vi "Acquire_Topology_Matrix.vi"(9 "All Path Array":string[](array[string]), 11 "Cluster of 7 Type Data":T2(array[cluster])) -> (2 "Topology Matrix":dbl[][](array[numeric]))   [LabVIEW 2014]
doc: "生成节点的拓扑矩阵"
uses:
  <vilib>/Analysis/Matrix/Datatypes/RealMatrix.ctl
  <vilib>/Analysis/Matrix/NI_Matrix.lvlib
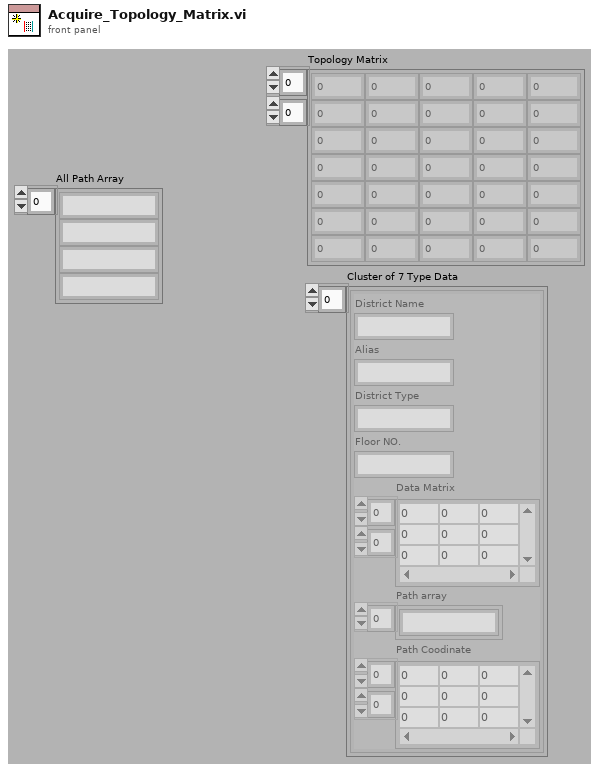
[diagram p1: front panel]
types:
  T1 = typedef "NI_Matrix.lvlib/RealMatrix.ctl" = dbl[][]
  T2 = cluster{"District Name":string, "Alias":string, "District Type":string, "Floor NO.":string, "Data Matrix":T1, "Path array":string[], "Path Coodinate":T1}[]
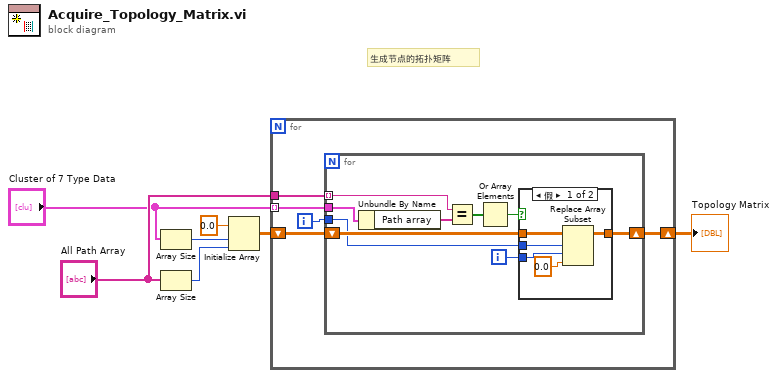
[diagram p0: block diagram]
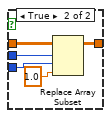
[diagram p2: hidden frame]
diagram:
  # "生成节点的拓扑矩阵"
  n1 = Array Size(array="Cluster of 7 Type Data") -> (size(s)=w5:i32)
  n2 = Array Size(array="All Path Array") -> (size(s)=w4:i32)
  n3 = Initialize Array(0.0 ("元素"), w5, w4) -> (w3:dbl[][])
  n4 = for {
    tunnel: "Cluster of 7 Type Data" -> [w11] mode=indexing
    tunnel: "All Path Array" -> [w12]
    shift-right: [w8] -> w7
    shift-left: w3 -> [w10]
    i -> [w9]
    n5 = for {
      tunnel: w12 -> [w19] mode=indexing
      tunnel: w11 -> [w21]
      tunnel: w9 -> [w16]
      shift-right: [w14] -> w8
      shift-left: w10 -> [w17]
      i -> [w15]
      n6 = Unbundle By Name(w21) -> ("Path array"=w20:string[])
      n7 = Equal?(x=w19, y=w20) -> (x = y?=w18:bool[])
      n8 = Or Array Elements(Boolean array=w18) -> (logical OR=w13:bool)
      n9 = case shown="假" w13 {
        tunnel: w17 -> [w25 w31]
        tunnel: w16 -> [w24 w30]
        tunnel: w15 -> [w23 w29]
        tunnel: [w22 w27] -> w14
        frame False {
          n10 = Replace Array Subset(array=w25, new element=0.0 ("新元素/子数组"), index (row)=w24, index (col)=w23) -> (w22:dbl[][])
        }
        frame True {
          n11 = Replace Array Subset(array=w31, new element=1.0 ("新元素/子数组"), index (row)=w30, index (col)=w29) -> (w27:dbl[][])
        }
      }
    }
  }
  "Topology Matrix" <- w7
